vi "write_ext_in.vi"(4 "power value":dbl, 5 "position num":u32, 6 "shutter en entrée":bool, 7 "pdir_path":path, 9 "shutter 1":bool, 10 "z value":dbl, 11 "chanel num":u8) -> (0 "sortie d'erreur":errorcluster)   [LabVIEW 2013]
panel:
  in  "power value 2":dbl
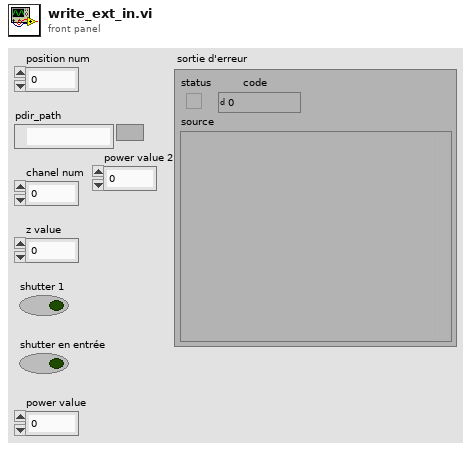
[diagram p1: front panel]
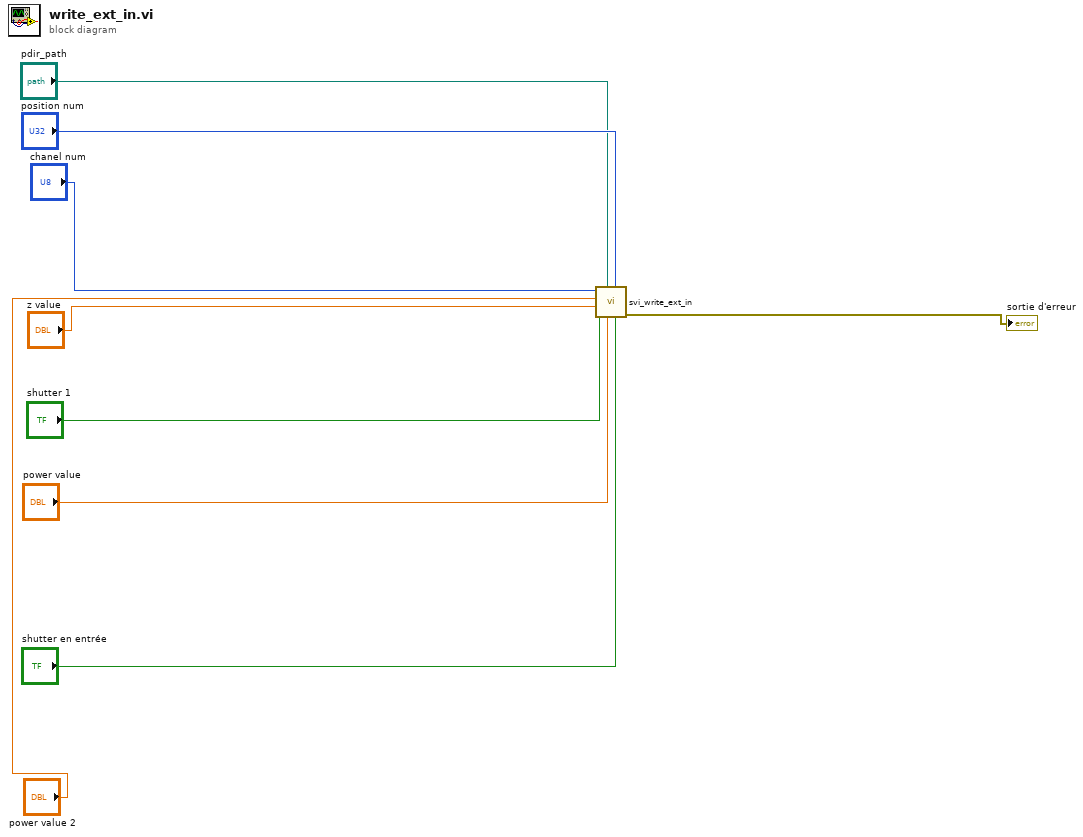
[diagram p0: block diagram]
diagram:
  n1 = call "svi_write_ext_in.vi"("shutter en entrée"="shutter en entrée", "position num"="position num", "power value"="power value", "pdir_path"="pdir_path", "shutter 1"="shutter 1", "z value"="z value", "power value 2"="power value 2", "chanel num"="chanel num") -> ("sortie d'erreur"=→"sortie d'erreur":errorcluster)  [unwired: 3 in]
